vi "Teleop.vi"(10 "Match Info":T1={"Autonomous Elapsed Seconds"=0.0, "TeleOp Elapsed Seconds"=0.0, "Disabled Elapsed Seconds"=0.0, "Visited Autonomous"=FALSE, "Visited TeleOp"=FALSE, "Visited Disabled"=FALSE, "Autonomous Settings"={"Autonomous Style"=enum."Independent", "VI Refnum"=refnum}}, 11 "Call Context":T2) -> ()   [LabVIEW 2019]
doc: "This VI is called for each enabled TeleOp packet received from the DS. It is typically used to read from joysticks and other inputs and update I/O or setpoints for timed control loops. It should complete and return within 20 milliseconds or risk missing DS packets."
uses:
  <vilib>/Rock Robotics/WPI/DriverStation/WPI_DriverStationDerivedRobotMode.ctl
  <vilib>/Rock Robotics/WPI/DriverStation/WPI_DriverStationMatch Info.ctl
  <vilib>/Rock Robotics/WPI/Solenoid/WPI_SolenoidValue.ctl
  Framework/Robot Global Data.vi
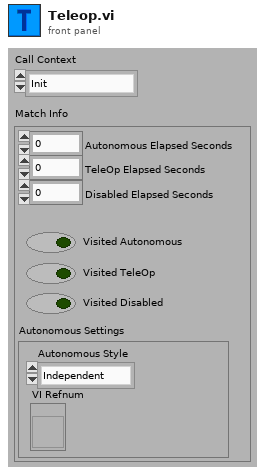
[diagram p1: front panel]
types:
  T1 = typedef "WPI_DriverStationMatch Info.ctl" = cluster{"Autonomous Elapsed Seconds":dbl, "TeleOp Elapsed Seconds":dbl, "Disabled Elapsed Seconds":dbl, "Visited Autonomous":bool, "Visited TeleOp":bool, "Visited Disabled":bool, "Autonomous Settings":cluster{"Autonomous Style":enum16{"Iterative", "Independent"}, "VI Refnum":refnum<vi>}}
  T2 = typedef "WPI_DriverStationDerivedRobotMode.ctl" = enum16{"Init", "Execute", "Stop"}
  T3 = typedef "WPI_SolenoidValue.ctl" = enum16{"Off", "On", "Forward", "Reverse"}
  T4 = typedef "Command Status Info.ctl" = cluster{"Name":string, "Status":T5, "notifier out":T6}
  T5 = typedef "Completion Status.ctl" = enum16{"Successful", "Aborted", "Incomplete"}
  T6 = typedef "Completion Notifier.ctl" = refnum<notifier>
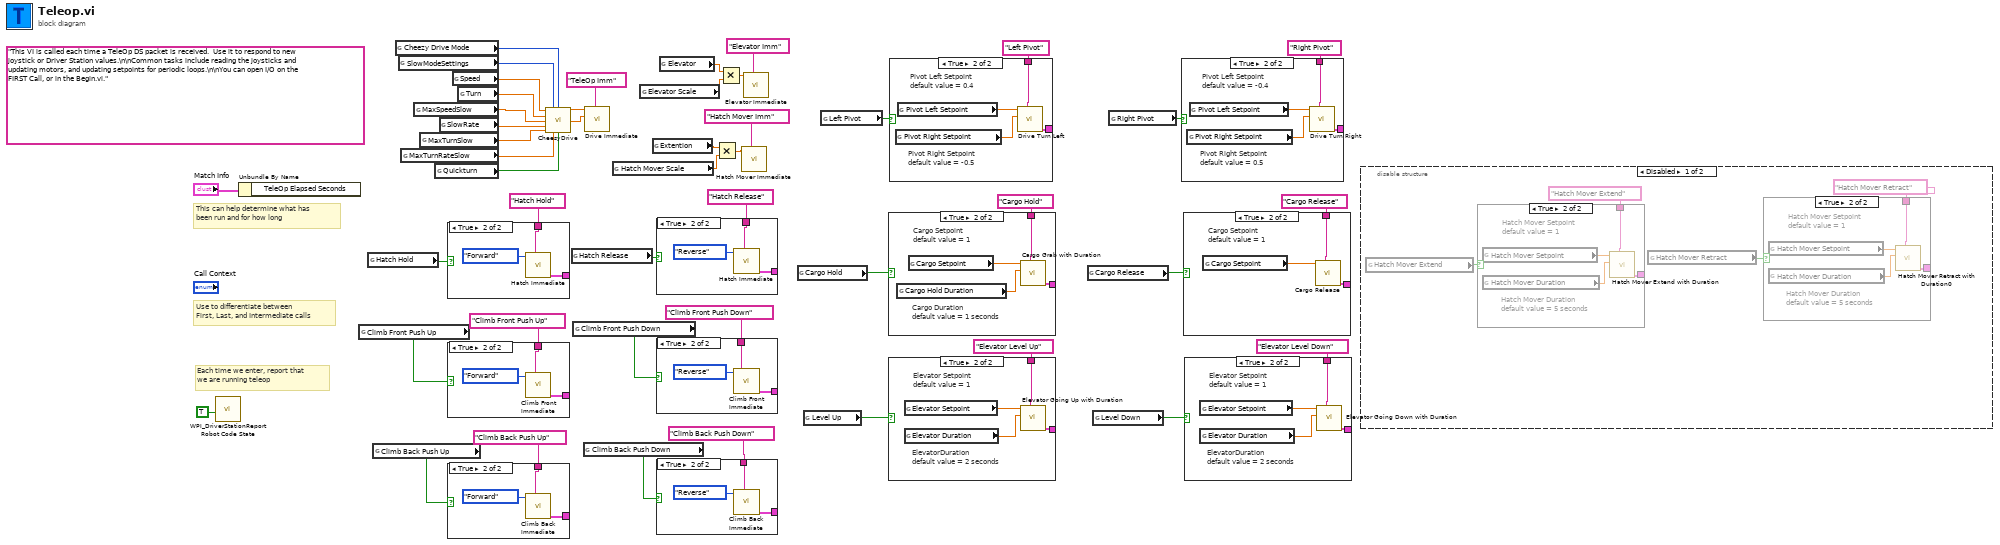
[diagram p0: block diagram]
diagram:
  (unwired) "This VI is called each time a TeleOp DS packet is received.  Use it to respond to new joystick or Driver Station values.\n\nCommon tasks include reading the joysticks and updating motors, and updating setpoints for periodic loops.\n\nYou can open I/O on the FIRST Call, or in the Begin.vi."
  # "Each time we enter, report that\nwe are running teleop"
  # "Use to differentiate between\nFirst, Last, and Intermediate calls"
  # "This can help determine what has\nbeen run and for how long"
  n1 = call <vilib>:"WPI_DriverStationReport Robot Code State.vi"("TeleOp"=TRUE ("Autonomous")) -> ()  [unwired: 10 in, 1 out]
  n2 = Unbundle By Name("Match Info") -> ()  [unwired: 1 out]
  n3 = global read "Robot Global Data.vi" "Climb Front Push Up"() -> (w38:bool)
  n4 = global read "Robot Global Data.vi" "Hatch Hold"() -> (w42:bool)
  n5 = global read "Robot Global Data.vi" "Climb Back Push Up"() -> (w35:bool)
  n6 = global read "Robot Global Data.vi" "Cheezy Drive Mode"() -> (w19:u32)
  n7 = global read "Robot Global Data.vi" "SlowModeSettings"() -> (w18:i32)
  n8 = global read "Robot Global Data.vi" "MaxTurnRateSlow"() -> (w12:dbl)
  n9 = global read "Robot Global Data.vi" "MaxSpeedSlow"() -> (w15:dbl)
  n10 = global read "Robot Global Data.vi" "MaxTurnSlow"() -> (w13:dbl)
  n11 = global read "Robot Global Data.vi" "Quickturn"() -> (w11:bool)
  n12 = global read "Robot Global Data.vi" "SlowRate"() -> (w14:dbl)
  n13 = case shown="True" w42 {
    tunnel: [_ w48] -> _
    tunnel: "Hatch Hold" ("Description") -> [_ w47]
    frame False {
    }
    frame True {
      n14 = call "Hatch Immediate.vi"("Description"=w47, "Action"=WPI_SolenoidValue."Forward") -> ("Command Info Out"=w48:T4)  [unwired: 9 in]
    }
  }
  n15 = case shown="True" w38 {
    tunnel: [_ w51] -> _
    tunnel: "Climb Front Push Up" ("Description") -> [_ w50]
    frame False {
    }
    frame True {
      n16 = call "Climb Front Immediate.vi"("Description"=w50, "Action"=WPI_SolenoidValue."Forward") -> ("Command Info Out"=w51:T4)  [unwired: 9 in]
    }
  }
  n17 = case shown="True" w35 {
    tunnel: [_ w55] -> _
    tunnel: "Climb Back Push Up" ("Description") -> [_ w54]
    frame False {
    }
    frame True {
      n18 = call "Climb Back Immediate.vi"("Description"=w54, "Relay Value"=WPI_SolenoidValue."Forward" ("Action")) -> ("Command Info Out"=w55:T4)  [unwired: 9 in]
    }
  }
  n19 = global read "Robot Global Data.vi" "Speed"() -> (w17:dbl)
  n20 = global read "Robot Global Data.vi" "Turn"() -> (w16:dbl)
  n21 = call "CheesyDrive.vi"("Throttle"=w17, "SlowModeSettings"=w18, "SlowMode"=w19, "Wheel"=w16, "MaxSpeedSlow"=w15, "SlowRate"=w14, "MaxTurnSlow"=w13, "MaxTurnRateSlow"=w12, "Quickturn"=w11) -> ("Left PWM"=w10:dbl, "Right PWM"=w9:dbl)  [unwired: 5 in]
  n22 = global read "Robot Global Data.vi" "Hatch Release"() -> (w41:bool)
  n23 = global read "Robot Global Data.vi" "Climb Front Push Down"() -> (w39:bool)
  n24 = global read "Robot Global Data.vi" "Climb Back Push Down"() -> (w34:bool)
  n25 = call "Drive Immediate.vi"("Description"="TeleOp Imm", "Right Setpoint"=w9, "Left Setpoint"=w10) -> ()  [unwired: 8 in, 1 out]
  n26 = global read "Robot Global Data.vi" "Hatch Mover Scale"() -> (w4:dbl)
  n27 = global read "Robot Global Data.vi" "Elevator Scale"() -> (w1:dbl)
  n28 = global read "Robot Global Data.vi" "Extention"() -> (w5:dbl)
  n29 = case shown="True" w41 {
    tunnel: [_ w57] -> _
    tunnel: "Hatch Release" ("Description") -> [_ w56]
    frame False {
    }
    frame True {
      n30 = call "Hatch Immediate.vi"("Description"=w56, "Action"=WPI_SolenoidValue."Reverse") -> ("Command Info Out"=w57:T4)  [unwired: 9 in]
    }
  }
  n31 = case shown="True" w39 {
    tunnel: [_ w60] -> _
    tunnel: "Climb Front Push Down" ("Description") -> [_ w59]
    frame False {
    }
    frame True {
      n32 = call "Climb Front Immediate.vi"("Description"=w59, "Action"=WPI_SolenoidValue."Reverse") -> ("Command Info Out"=w60:T4)  [unwired: 9 in]
    }
  }
  n33 = case shown="True" w34 {
    tunnel: [_ w64] -> _
    tunnel: "Climb Back Push Down" ("Description") -> [_ w63]
    frame False {
    }
    frame True {
      n34 = call "Climb Back Immediate.vi"("Description"=w63, "Relay Value"=WPI_SolenoidValue."Reverse" ("Action")) -> ("Command Info Out"=w64:T4)  [unwired: 9 in]
    }
  }
  n35 = global read "Robot Global Data.vi" "Elevator"() -> (w2:dbl)
  n36 = Multiply(x=w5, y=w4) -> (x*y=w6:dbl)
  n37 = Multiply(x=w2, y=w1) -> (x*y=w3:dbl)
  n38 = call "Hatch Mover Immediate.vi"("Description"="Hatch Mover Imm", "Setpoint"=w6) -> ()  [unwired: 9 in, 1 out]
  n39 = call "Elevator Immediate.vi"("Description"="Elevator Imm", "Setpoint"=w3) -> ()  [unwired: 9 in, 1 out]
  n40 = global read "Robot Global Data.vi" "Cargo Hold"() -> (w26:bool)
  n41 = global read "Robot Global Data.vi" "Level Up"() -> (w23:bool)
  n42 = global read "Robot Global Data.vi" "Left Pivot"() -> (w30:bool)
  n43 = case shown="True" w26 {
    tunnel: "Cargo Hold" ("Description") -> [_ w68]
    tunnel: [_ w65] -> _
    frame False {
    }
    frame True {
      # "Cargo Duration\ndefault value = 1 seconds"
      # "Cargo Setpoint\ndefault value = 1"
      n44 = global read "Robot Global Data.vi" "Cargo Hold Duration"() -> (w66:dbl)
      n45 = global read "Robot Global Data.vi" "Cargo Setpoint"() -> (w67:dbl)
      n46 = call "Cargo Grab with Duration.vi"("Description"=w68, "Duration (s)"=w66, "Setpoint"=w67) -> ("Command Info Out"=w65:T4)  [unwired: 8 in]
    }
  }
  n47 = case shown="True" w23 {
    tunnel: "Elevator Level Up" ("Description") -> [_ w72]
    tunnel: [_ w69] -> _
    frame False {
    }
    frame True {
      # "ElevatorDuration\ndefault value = 2 seconds"
      # "Elevator Setpoint\ndefault value = 1"
      n48 = global read "Robot Global Data.vi" "Elevator Setpoint"() -> (w71:dbl)
      n49 = global read "Robot Global Data.vi" "Elevator Duration"() -> (w70:dbl)
      n50 = call "Elevator Going Up with Duration.vi"("Description"=w72, "Duration (s)"=w70, "Setpoint"=w71) -> ("Command Info Out"=w69:T4)  [unwired: 8 in]
    }
  }
  n51 = case shown="True" w30 {
    tunnel: "Left Pivot" ("Description") -> [_ w76]
    tunnel: [_ w73] -> _
    frame False {
    }
    frame True {
      # "Pivot Right Setpoint\ndefault value = -0.5"
      # "Pivot Left Setpoint\ndefault value = 0.4"
      n52 = global read "Robot Global Data.vi" "Pivot Right Setpoint"() -> (w74:dbl)
      n53 = global read "Robot Global Data.vi" "Pivot Left Setpoint"() -> (w75:dbl)
      n54 = call "Drive Turn Left.vi"("Description"=w76, "Right Setpoint"=w74, "Left Setpoint"=w75) -> ("Command Info Out"=w73:T4)  [unwired: 8 in]
    }
  }
  n55 = global read "Robot Global Data.vi" "Cargo Release"() -> (w25:bool)
  n56 = global read "Robot Global Data.vi" "Level Down"() -> (w20:bool)
  n57 = global read "Robot Global Data.vi" "Right Pivot"() -> (w29:bool)
  n58 = case shown="True" w29 {
    tunnel: "Right Pivot" ("Description") -> [_ w80]
    tunnel: [_ w77] -> _
    frame False {
    }
    frame True {
      # "Pivot Right Setpoint\ndefault value = 0.5"
      # "Pivot Left Setpoint\ndefault value = -0.4"
      n59 = global read "Robot Global Data.vi" "Pivot Right Setpoint"() -> (w78:dbl)
      n60 = global read "Robot Global Data.vi" "Pivot Left Setpoint"() -> (w79:dbl)
      n61 = call "Drive Turn Right.vi"("Description"=w80, "Right Setpoint"=w78, "Left Setpoint"=w79) -> ("Command Info Out"=w77:T4)  [unwired: 8 in]
    }
  }
  n62 = case shown="True" w25 {
    tunnel: "Cargo Release" ("Description") -> [_ w83]
    tunnel: [_ w81] -> _
    frame False {
    }
    frame True {
      # "Cargo Setpoint\ndefault value = 1"
      n63 = global read "Robot Global Data.vi" "Cargo Setpoint"() -> (w82:dbl)
      n64 = call "Cargo Release.vi"("Description"=w83, "Setpoint"=w82) -> ("Command Info Out"=w81:T4)  [unwired: 9 in]
    }
  }
  n65 = case shown="True" w20 {
    tunnel: "Elevator Level Down" ("Description") -> [_ w87]
    tunnel: [_ w84] -> _
    frame False {
    }
    frame True {
      # "ElevatorDuration\ndefault value = 2 seconds"
      # "Elevator Setpoint\ndefault value = 1"
      n66 = global read "Robot Global Data.vi" "Elevator Setpoint"() -> (w86:dbl)
      n67 = global read "Robot Global Data.vi" "Elevator Duration"() -> (w85:dbl)
      n68 = call "Elevator Going Down with Duration.vi"("Description"=w87, "Duration (s)"=w85, "Setpoint"=w86) -> ("Command Info Out"=w84:T4)  [unwired: 8 in]
    }
  }
  n69 = disable-structure shown="Disabled" {
    frame Disabled {
      n70 = global read "Robot Global Data.vi" "Hatch Mover Extend"() -> (w89:bool)
      n71 = case shown="True" w89 {
        tunnel: "Hatch Mover Extend" ("Description") -> [_ w95]
        tunnel: [_ w92] -> _
        frame False {
        }
        frame True {
          # "Hatch Mover Duration\ndefault value = 5 seconds"
          # "Hatch Mover Setpoint\ndefault value = 1"
          n72 = global read "Robot Global Data.vi" "Hatch Mover Setpoint"() -> (w94:dbl)
          n73 = global read "Robot Global Data.vi" "Hatch Mover Duration"() -> (w93:dbl)
          n74 = call "Hatch Mover Extend with Duration.vi"("Description"=w95, "Duration (s)"=w93, "Setpoint"=w94) -> ("Command Info Out"=w92:T4)  [unwired: 8 in]
        }
      }
      n75 = global read "Robot Global Data.vi" "Hatch Mover Retract"() -> (w91:bool)
      n76 = case shown="True" w91 {
        tunnel: "Hatch Mover Retract" ("Description") -> [_ w99]
        tunnel: [_ w96] -> _
        frame False {
        }
        frame True {
          # "Hatch Mover Duration\ndefault value = 5 seconds"
          # "Hatch Mover Setpoint\ndefault value = 1"
          n77 = global read "Robot Global Data.vi" "Hatch Mover Setpoint"() -> (w98:dbl)
          n78 = global read "Robot Global Data.vi" "Hatch Mover Duration"() -> (w97:dbl)
          n79 = call "Hatch Mover Retract with Duration0.vi"("Description"=w99, "Duration (s)"=w97, "Setpoint"=w98) -> ("Command Info Out"=w96:T4)  [unwired: 8 in]
        }
      }
    }
    frame Enabled {
    }
  }
